vi "Convert Callback Option.vi"(11 "Callback Option":T1) -> (3 "Callback Option String":string)   [LabVIEW 2011, in "Tinkerforge.lvlib" / "Device.lvclass"]
doc: "This VI converts the Callback Option enumeration to the protocol char."
uses:
  Device.lvclass
  Type Definitions/Callback Option.ctl
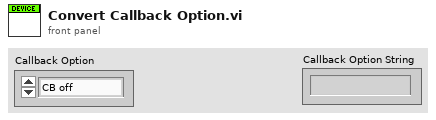
[diagram p1: front panel]
types:
  T1 = typedef "Tinkerforge.lvlib/Device.lvclass/Callback Option.ctl" = enum8{"CB off", "outside range", "inside range", "smaller", "greater"}
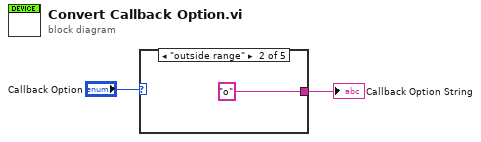
[diagram p0: block diagram]
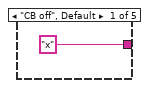
[diagram p2: hidden frame]
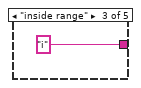
[diagram p3: hidden frame]
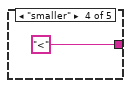
[diagram p4: hidden frame]
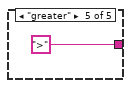
[diagram p5: hidden frame]
diagram:
  n1 = case shown="\"outside range\"" "Callback Option" {
    tunnel: ["x" "o" "i" "<" ">"] -> w1
    frame "CB off", Default {
    }
    frame "outside range" {
    }
    frame "inside range" {
    }
    frame "smaller" {
    }
    frame "greater" {
    }
  }
  "Callback Option String" <- w1
